vi "massive.vi"() -> ()   [LabVIEW 2021]
panel:
  out "element":dbl
  out "Numeric 2":dbl
  out "Numeric":dbl
  in  "Array 4":dbl[](array[numeric])
  out "appended array 2":dbl[](array[numeric])
  out "appended array":dbl[](array[numeric])
  in  "Array 3":dbl[](array[numeric])
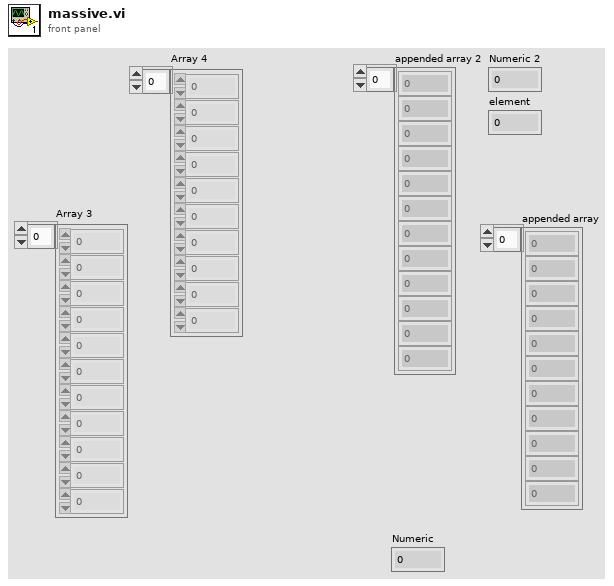
[diagram p1: front panel]
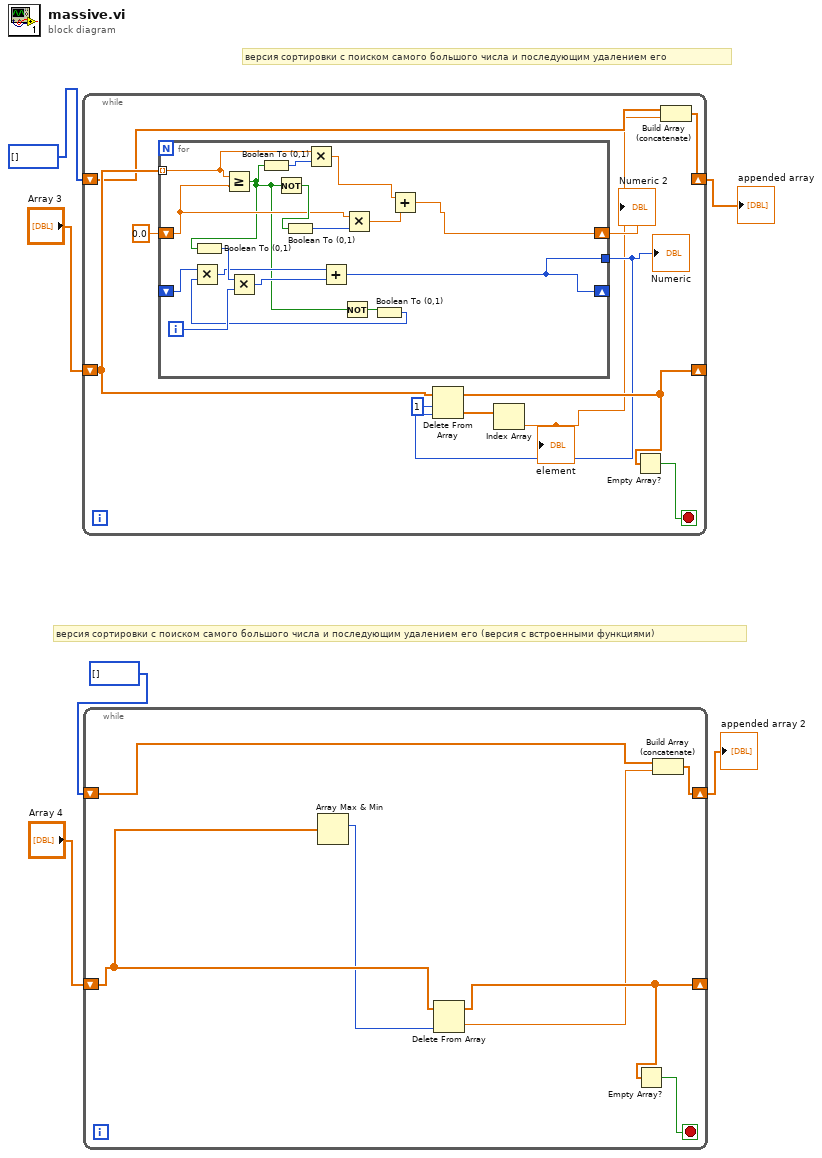
[diagram p0: block diagram]
diagram:
  # "версия сортировки с поиском самого большого числа и последующим удалением его (версия с встроенными функциями)"
  # "версия сортировки с поиском самого большого числа и последующим удалением его"
  n1 = while {
    shift-right: [w16] -> _
    shift-left: "Array 3" -> [w17]
    shift-right: [w14] -> w5
    shift-left: i32[] [] -> [w13]
    stop <- w15 stop-if-true
    n2 = for {
      tunnel: w17 -> [w28] mode=indexing
      shift-right: [w18] -> w11
      shift-left: 0.0 -> [w29]
      shift-right: [w24] -> _
      shift-left: _ -> [w23]
      tunnel: [w24] -> w12
      i -> [w27]
      n3 = Greater Or Equal?(x=w28, y=w29) -> (x >= y?=w21:bool)
      n4 = Boolean To (0,1)(Boolean=w21) -> (0, 1=w26:i16)
      n5 = Multiply(x=w26, y=w27) -> (x*y=w25:i32)
      n6 = Boolean To (0,1)(Boolean=w21) -> (0, 1=w31:i16)
      n7 = Not(x=w21) -> (.not. x?=w32:bool)
      n8 = Boolean To (0,1)(Boolean=w32) -> (0, 1=w30:i16)
      n9 = Multiply(x=w28, y=w31) -> (x*y=w34:dbl)
      n10 = Not(x=w21) -> (.not. x?=w20:bool)
      n11 = Multiply(x=w29, y=w30) -> (x*y=w33:dbl)
      n12 = Boolean To (0,1)(Boolean=w20) -> (0, 1=w19:i16)
      n13 = Multiply(x=w23, y=w19) -> (x*y=w22:i32)
      n14 = Add(x=w22, y=w25) -> (x+y=w24:i32)
      n15 = Add(x=w34, y=w33) -> (x+y=w18:dbl)
    }
    "Numeric" <- w12
    "Numeric 2" <- w11
    n16 = Delete From Array(array=w17, length=1, index=w12) -> (deleted portion=w9:dbl[], array with subset deleted=w16:dbl[])
    n17 = Index Array(array=w9) -> (element=w8:dbl)  [unwired: 1 in]
    "element" <- w8
    n18 = Empty Array?(array=w16) -> (empty?=w15:bool)
    n19 = Build Array (concatenate)(w13, w8) -> (w14:dbl[])
  }
  "appended array" <- w5
  n20 = while {
    shift-right: [w41] -> _
    shift-left: "Array 4" -> [w36]
    shift-right: [w38] -> w2
    shift-left: i32[] [] -> [w37]
    stop <- w40 stop-if-true
    n21 = Array Max & Min(array=w36) -> (max index (indices)=w35:i32)  [unwired: 3 out]
    n22 = Delete From Array(array=w36, index=w35) -> (deleted portion=w39:dbl, array with subset deleted=w41:dbl[])  [unwired: 1 in]
    n23 = Empty Array?(array=w41) -> (empty?=w40:bool)
    n24 = Build Array (concatenate)(w37, w39) -> (w38:dbl[])
  }
  "appended array 2" <- w2
